vi "Read currentAtmosphericDispersion_arcsec.vi"(8 "error in (no error)":errorcluster, 11 "TCSAtmosphericDispersionStatus in":refnum<class "TCSAtmosphericDispersionStatus.lvclass">) -> (0 "error out":errorcluster, 2 "currentAtmosphericDispersion_arcsec":dbl[unit] min=-0.00048481368110953597 max=0.00048481368110953597, 3 "TCSAtmosphericDispersionStatus out":refnum<class "TCSAtmosphericDispersionStatus.lvclass">)   [LabVIEW 2022 SP3, in "TCSDataDefinitions.lvlib" / "TCSAtmosphericDispersionStatus.lvlib" / "TCSAtmosphericDispersionStatus.lvclass"]
uses:
  TCSAtmosphericDispersionStatus.lvclass
  TCSAtmosphericDispersionStatus.lvclass/TCSAtmosphericDispersionStatus.ctl
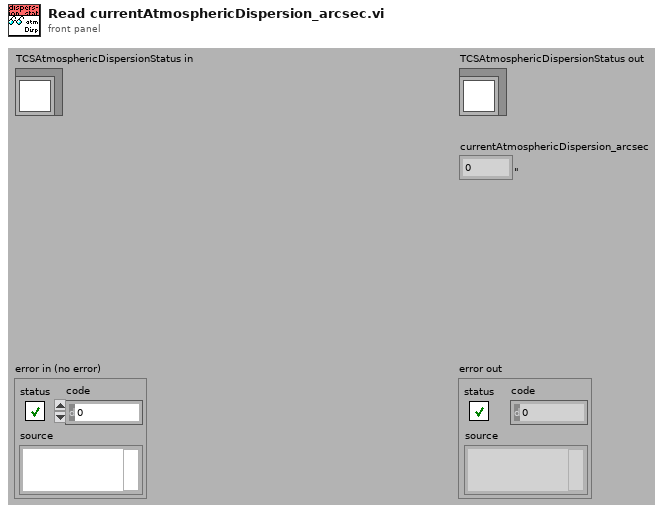
[diagram p1: front panel]
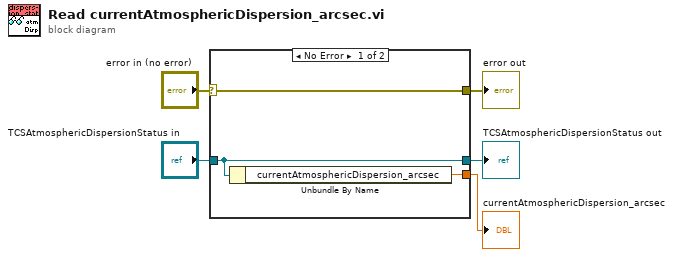
[diagram p0: block diagram]
diagram:
  n1 = case shown="No Error" "error in (no error)" {
    selector: "error in (no error)" -> [w8 w9]
    tunnel: [w8 w9] -> w4
    tunnel: [w7 w10] -> w2
    tunnel: "TCSAtmosphericDispersionStatus in" -> [w7 w10]
    tunnel: [w6 _] -> w1
    frame No Error {
      n2 = Unbundle By Name(w7) -> ("currentAtmosphericDispersion_arcsec"=w6:dbl[unit])
    }
    frame Error {
    }
  }
  "error out" <- w4
  "TCSAtmosphericDispersionStatus out" <- w2
  "currentAtmosphericDispersion_arcsec" <- w1
